vi "lock-in input sweep - T dependent.vi"() -> ()   [LabVIEW 2022 SP3]
uses:
  <vilib>/Utility/file.llb/Write To Spreadsheet File (DBL).vi
panel:
  out "phase":dbl=-1.07289e-06
  in  "Parameter (1: X) 2":u16(ring)=2 items=["X"=1, "Y"=2, "R"=3, "Theta"=4, "Channel 1"=5, "Channel 2"=6, "Aux In 1"=7, "Aux In 2"=8, "Aux In 3"=9, "Aux In 4"=10]
  in  "auto phase":bool
  in  "manual phase":dbl
  in  "harm#2":dbl=1.0
  out "loop run":i32=1
  in  "loop #":i32=1
  in  "Save data or not":bool=TRUE
  in  "path (folder + filename)":string="D:\\test"
  in  "Clear Plot":bool
  out "XY Graph":cluster{dbl[], dbl[]}(graph)={[0.0, 0.020000000000000018, 0.040000000000000036, 0.05999999999999994, 0.07999999999999996, 0.09999999999999998, 0.12, 0.14, 0.16000000000000003, 0.17999999999999994, 0.19999999999999996, 0.21999999999999997, 0.24, 0.26, 0.28, 0.29999999999999993, 0.31999999999999995, 0.33999999999999997, 0.36, 0.38, 0.4, 0.42000000000000004, 0.43999999999999995, 0.45999999999999996, 0.48, 0.5, 0.52, 0.54, 0.56, 0.5800000000000001, 0.6, 0.62, 0.64, 0.6599999999999999, 0.6799999999999999, 0.7, 0.72, 0.74, 0.76, 0.78, 0.8, 0.8200000000000001, 0.84, 0.86, 0.88, 0.9, 0.92, 0.94, 0.96, 0.98, 1.0, 0.98, 0.96, 0.94, 0.9199999999999999, 0.9000000000000001, 0.8800000000000001, 0.8600000000000001, 0.8400000000000001, 0.8200000000000001, 0.8, 0.78, 0.76, 0.74, 0.72, 0.7, 0.6799999999999999, 0.6600000000000001, 0.6400000000000001, 0.6200000000000001, 0.6000000000000001, 0.5800000000000001, 0.56, 0.54, 0.52, 0.5, 0.48, 0.45999999999999996, 0.43999999999999995, 0.41999999999999993, 0.40000000000000013, 0.3800000000000001, 0.3600000000000001, 0.3400000000000001, 0.32000000000000006, 0.30000000000000004, 0.28, 0.26, 0.24, 0.21999999999999997, 0.19999999999999996, 0.17999999999999994, 0.15999999999999992, 0.14000000000000012, 0.1200000000000001, 0.10000000000000009, 0.08000000000000007, 0.06000000000000005, 0.040000000000000036, 0.020000000000000018, 0.0, 0.020000000000000018, 0.040000000000000036, 0.05999999999999994, 0.07999999999999996, 0.09999999999999998, 0.12, 0.14, 0.16000000000000003, 0.17999999999999994, 0.19999999999999996, 0.21999999999999997, 0.24, 0.26, 0.28, 0.29999999999999993, 0.31999999999999995, 0.33999999999999997, 0.36, 0.38, 0.4, 0.42000000000000004, 0.43999999999999995, 0.45999999999999996, 0.48, 0.5, 0.52, 0.54, 0.56, 0.5800000000000001, 0.6, 0.62, 0.64, 0.6599999999999999, 0.6799999999999999, 0.7, 0.72, 0.74, 0.76, 0.78, 0.8, 0.8200000000000001, 0.84, 0.86, 0.88, 0.9, 0.92, 0.94, 0.96, 0.98, 1.0, 0.98, 0.96, 0.9400000000000001, 0.92, 0.9, 0.88, 0.86, 0.84, 0.8200000000000001, 0.8, 0.78, 0.76, 0.74, 0.72, 0.7000000000000001, 0.68, 0.66, 0.64, 0.62, 0.6, 0.58, 0.56, 0.54, 0.52, 0.5, 0.48, 0.46, 0.44, 0.42, 0.4, 0.38, 0.36, 0.34, 0.32, 0.3, 0.28, 0.26, 0.24, 0.22, 0.2, 0.18, 0.16, 0.14, 0.12, 0.1, 0.08, 0.06, 0.04, 0.02, 0.0, 0.0, 0.19999999999999996, 0.3999999999999999, 0.6, 0.8, 1.0, 0.8, 0.6000000000000001, 0.40000000000000013, 0.20000000000000018, 0.0, 0.19999999999999996, 0.3999999999999999, 0.6, 0.8, 1.0, 0.8, 0.6000000000000001, 0.4, 0.2, 0.0, 0.0, 0.19999999999999996, 0.3999999999999999, 0.6, 0.8, 1.0, 0.8, 0.6000000000000001, 0.40000000000000013, 0.20000000000000018, 0.0, 0.19999999999999996, 0.3999999999999999, 0.6, 0.8, 1.0, 0.8, 0.6000000000000001, 0.4, 0.2, 0.0, 0.0], [-2.3842e-07, -3.5763e-07, -2.3842e-07, -1.1921e-07, 0.0, 0.0, 0.0, 1.1921e-07, 1.1921e-07, 3.5763e-07, 5.9605e-07, 5.9605e-07, 5.9605e-07, 4.76841e-07, 3.5763e-07, 1.1921e-07, 1.1921e-07, 1.1921e-07, 3.5763e-07, 3.5763e-07, 2.3842e-07, 1.1921e-07, -1.1921e-07, -3.5763e-07, -5.9605e-07, -4.76841e-07, -3.5763e-07, -2.3842e-07, 0.0, 0.0, 0.0, -2.3842e-07, -2.3842e-07, -1.1921e-07, -2.3842e-07, -2.3842e-07, -2.3842e-07, -2.3842e-07, -3.5763e-07, -2.3842e-07, -2.3842e-07, -2.3842e-07, -3.5763e-07, -2.3842e-07, -1.1921e-07, 0.0, 1.1921e-07, 0.0, 0.0, -1.1921e-07, -1.1921e-07, 0.0, 0.0, 0.0, 0.0, 0.0, 0.0, 0.0, -1.1921e-07, -2.3842e-07, -3.5763e-07, -3.5763e-07, -3.5763e-07, -2.3842e-07, -2.3842e-07, 0.0, 2.3842e-07, 3.5763e-07, 3.5763e-07, 2.3842e-07, 2.3842e-07, 2.3842e-07, 3.5763e-07, 5.9605e-07, 5.9605e-07, 7.15259e-07, 8.34469e-07, 8.34469e-07, 5.9605e-07, 1.1921e-07, -1.1921e-07, -2.3842e-07, -2.3842e-07, -1.1921e-07, 0.0, 1.1921e-07, 1.1921e-07, 0.0, 0.0, 1.1921e-07, 2.3842e-07, 3.5763e-07, 3.5763e-07, 2.3842e-07, 2.3842e-07, 1.1921e-07, -1.1921e-07, -2.3842e-07, -3.5763e-07, -4.76841e-07, -4.76841e-07, -4.76841e-07, -3.5763e-07, -3.5763e-07, -2.3842e-07, -2.3842e-07, -1.1921e-07, 0.0, 1.1921e-07, 2.3842e-07, 3.5763e-07, 2.3842e-07, 0.0, -2.3842e-07, -3.5763e-07, -3.5763e-07, -3.5763e-07, -2.3842e-07, -1.1921e-07, -1.1921e-07, 0.0, 1.1921e-07, 1.1921e-07, 1.1921e-07, 0.0, 0.0, -1.1921e-07, 0.0, -1.1921e-07, -1.1921e-07, -1.1921e-07, -1.1921e-07, -2.3842e-07, -1.1921e-07, 1.1921e-07, 2.3842e-07, 1.1921e-07, 0.0, -1.1921e-07, -3.5763e-07, -3.5763e-07, -3.5763e-07, -2.3842e-07, -2.3842e-07, 0.0, 1.1921e-07, 2.3842e-07, 2.3842e-07, 1.1921e-07, -1.1921e-07, -2.3842e-07, -3.5763e-07, -4.76841e-07, -7.15259e-07, -7.15259e-07, -7.15259e-07, -7.15259e-07, -4.76841e-07, -2.3842e-07, -2.3842e-07, -2.3842e-07, -3.5763e-07, -4.76841e-07, -4.76841e-07, -4.76841e-07, -3.5763e-07, -3.5763e-07, -2.3842e-07, -1.1921e-07, 1.1921e-07, 2.3842e-07, 3.5763e-07, 4.76841e-07, 5.9605e-07, 7.15259e-07, 7.15259e-07, 7.15259e-07, 5.9605e-07, 1.1921e-07, -1.1921e-07, -2.3842e-07, -2.3842e-07, -2.3842e-07, -2.3842e-07, -2.3842e-07, 0.0, 1.1921e-07, 2.3842e-07, 1.1921e-07, 0.0, -2.3842e-07, -2.3842e-07, -2.3842e-07, -2.3842e-07, -1.1921e-07, 0.0, -1.1921e-07, -1.1921e-07, -1.1921e-07, 0.0, 1.1921e-07, -2.3842e-07, -2.3842e-07, -2.3842e-07, -2.3842e-07, -2.3842e-07, -1.1921e-07, -1.1921e-07, 0.0, 0.0, 1.1921e-07, 1.1921e-07, 2.3842e-07, 2.3842e-07, 2.3842e-07, 2.3842e-07, 1.1921e-07, 0.0, -2.3842e-07, -2.3842e-07, -2.3842e-07, -2.3842e-07, -1.1921e-07, -1.1921e-07, -1.1921e-07, -2.3842e-07, -2.3842e-07, -3.5763e-07, -3.5763e-07, -4.76841e-07, -4.76841e-07, -4.76841e-07, -4.76841e-07, -4.76841e-07, -4.76841e-07, -4.76841e-07, -3.5763e-07, -3.5763e-07, -2.3842e-07, 0.0, 0.0, 1.1921e-07, 1.1921e-07, -4.76841e-07]}
  out "para1 Measurement":dbl=-2.3842e-07
  in  "Parameter (1: X)":u16(ring)=1 items=["X"=1, "Y"=2, "R"=3, "Theta"=4, "Channel 1"=5, "Channel 2"=6, "Aux In 1"=7, "Aux In 2"=8, "Aux In 3"=9, "Aux In 4"=10]
  out "gate voltage":dbl format="%#_13g"
  in  "GATE STEP(mv)":i32=20
  in  "GATE Low Value (default 0)":dbl
  in  "GATE High Value":dbl=1.0
  in  "lovkin waiting":dbl=0.2 format="%#_13g"
  in  "frequency":dbl=50.0 format="%#_13g"
  in  "Input Connection (0: Single-Ended Voltage)":u16(ring)=1 items=["Single-Ended Voltage", "Differential Voltage", "1 MOhm Current Gain", "100 MOhm Current Gain"]
  in  "LOCKIN address":refnum<visa-resource-name>="GPIB0::10::INSTR"
  # "Lock-in"
  # "top Gate Setting"
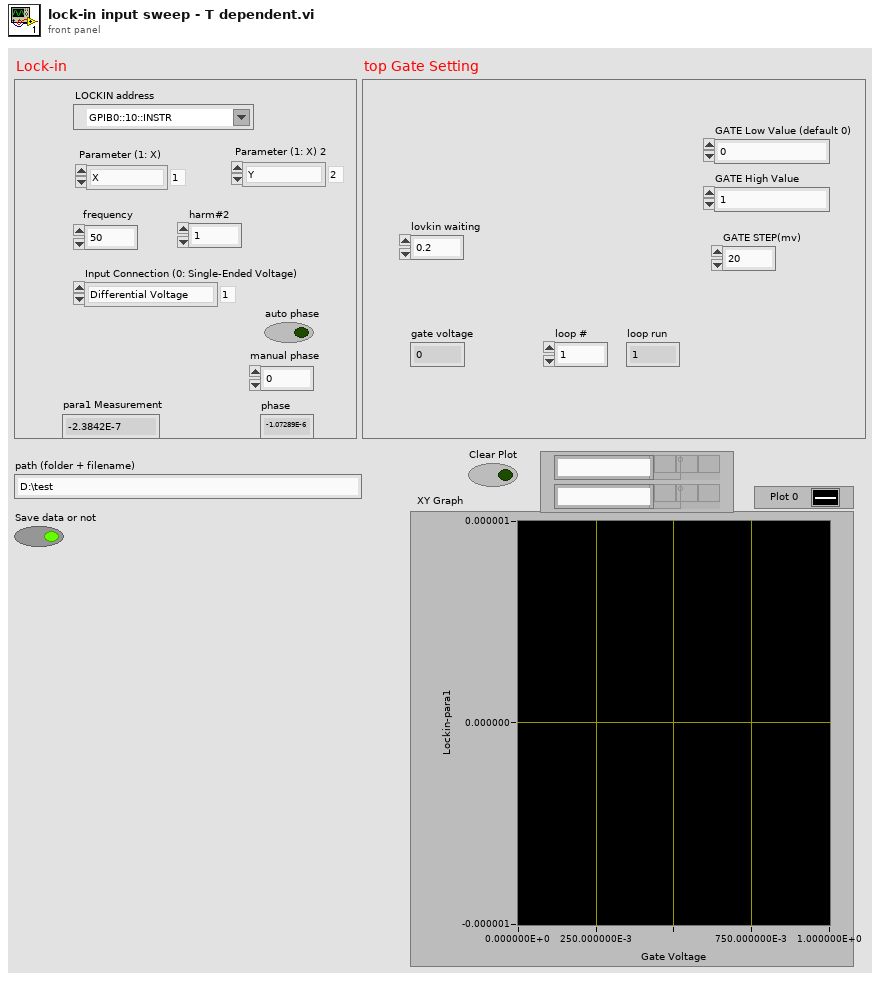
[diagram p1: front panel]
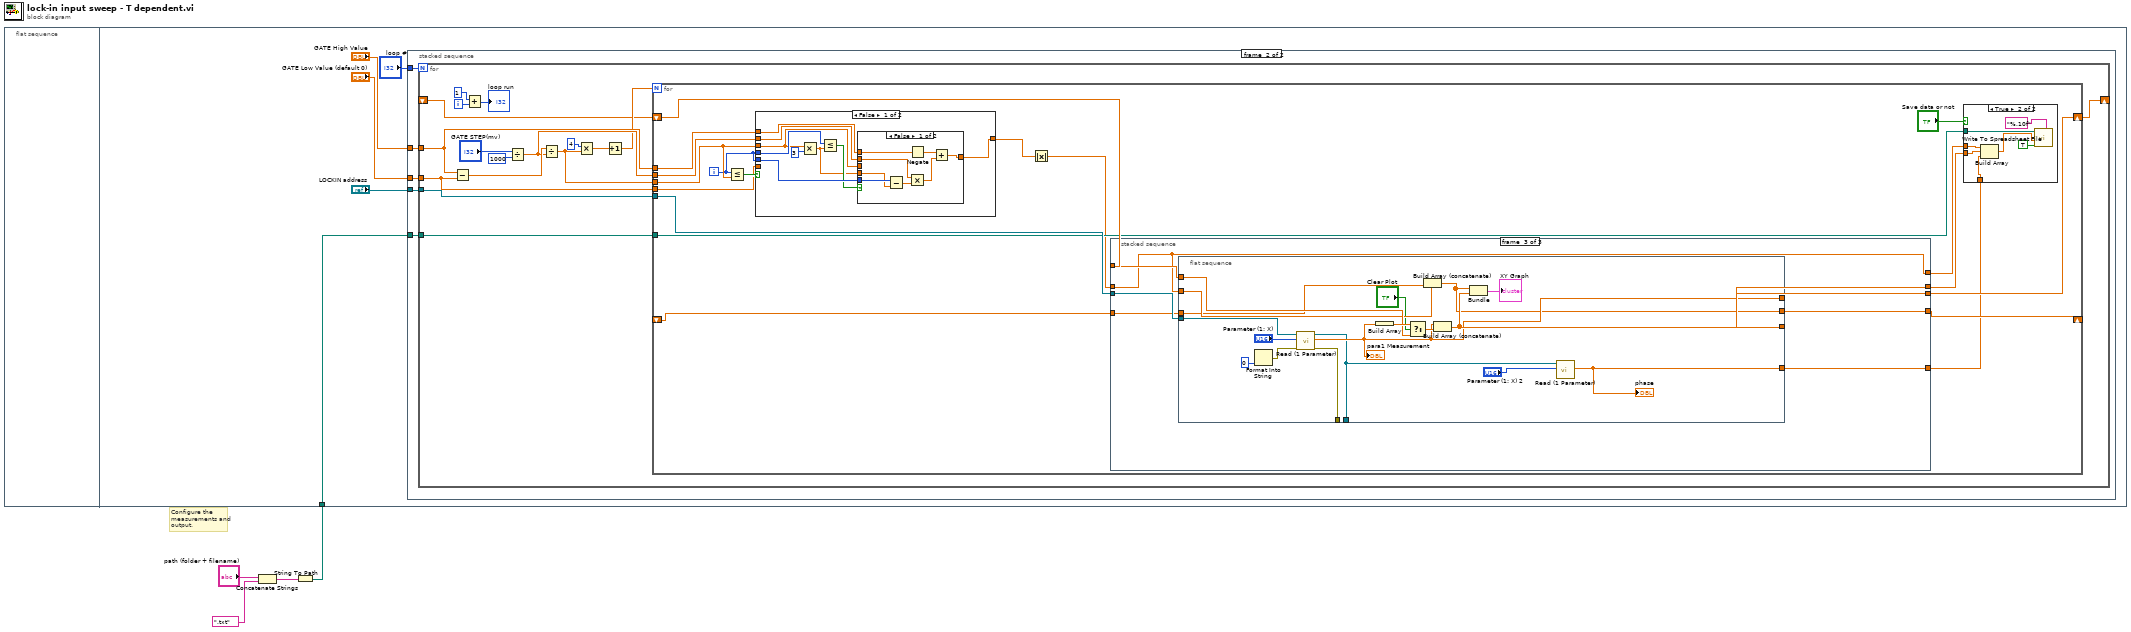
[diagram p0: block diagram]
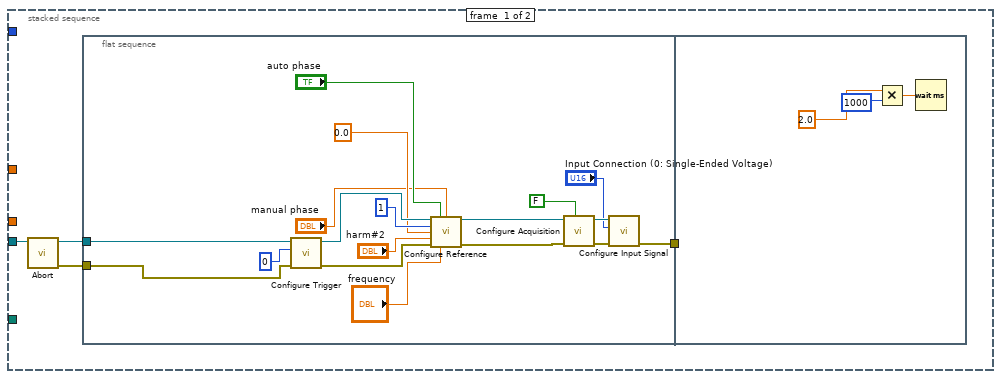
[diagram p2: hidden frame]
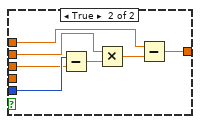
[diagram p4: hidden frame]
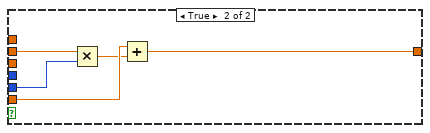
[diagram p5: hidden frame]
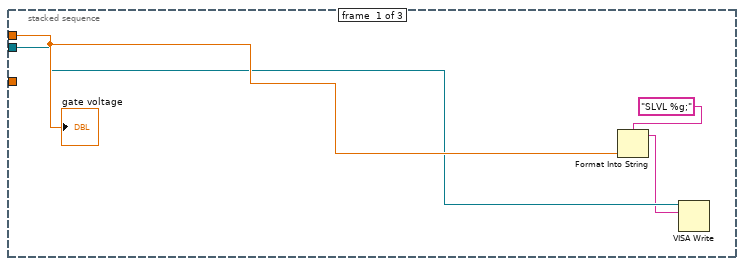
[diagram p6: hidden frame]
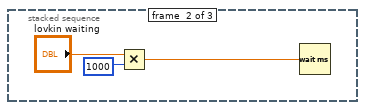
[diagram p7: hidden frame]
diagram:
  # "Configure the measurements and output."
  n1 = flat-sequence {
    tunnel: w1 -> [w6]
    frame #0 {
    }
    frame #1 {
      n2 = stacked-sequence {
        tunnel: "LOCKIN address" -> [w12 w39]
        tunnel: "GATE High Value" -> [_ w37]
        tunnel: "GATE Low Value (default 0)" -> [_ w38]
        tunnel: w6 -> [_ w36]
        tunnel: "loop #" -> [_ w35]
        frame #0 {
          n3 = call <instrlib>:"Abort.vi"("VISA resource name"=w12) -> ("error out"=w10:errorcluster, "VISA resource name out"=w11:refnum<visa-resource-name>)  [unwired: 9 in]
          n4 = flat-sequence {
            tunnel: w11 -> [w31]
            tunnel: [w16] -> w13
            tunnel: w10 -> [w15]
            tunnel: w13 -> [_]
            frame #0 {
              n5 = call <instrlib>:"Configure Trigger.vi"("error in (no error)"=w15, "Trigger Source (0: Internal)"=0, "VISA resource name"=w31) -> ("error out"=w25:errorcluster, "VISA resource name out"=w26:refnum<visa-resource-name>)  [unwired: 7 in]
              n6 = call <instrlib>:"Configure Reference.vi"("VISA resource name"=w26, "Auto Phase (T: Enabled)"="auto phase", "Manual Phase (0 Degree)"="manual phase", "Reference Source (1: Internal)"=1, "Sine Output Amplitude (1 V)"=0.0 ("Sine Output Amplitude (1 V) 2"), "Detection Harmonic Number (1)"="harm#2", "error in (no error)"=w25, "Internal Reference Frequency (1000 Hz)"="frequency") -> ("VISA resource name out"=w23:refnum<visa-resource-name>, "error out"=w18:errorcluster)  [unwired: 6 in]
              n7 = call <instrlib>:"Configure Acquisition.vi"("Continuous Storage (T: Enable)"=FALSE, "error in (no error)"=w18, "VISA resource name"=w23) -> ("error out"=w17:errorcluster, "VISA resource name out"=w21:refnum<visa-resource-name>)  [unwired: 7 in]
              n8 = call <instrlib>:"Configure Input Signal.vi"("error in (no error)"=w17, "Input Connection (0: Single-Ended Voltage)"="Input Connection (0: Single-Ended Voltage)", "VISA resource name"=w21) -> ("error out"=w16:errorcluster)  [unwired: 7 in, 1 out]
            }
            frame #1 {
              n9 = Multiply(x=2.0 ("SD stabilization(S) 2"), y=1000) -> (x*y=w34:dbl)
              n10 = Wait (ms)(milliseconds to wait=w34) -> ()  [unwired: 1 out]
            }
          }
        }
        frame #1 {
          n11 = for {
            N: w35 -> [_]
            tunnel: w39 -> [w56]
            tunnel: w38 -> [w50]
            tunnel: w37 -> [w49]
            tunnel: w36 -> [w48]
            shift-right: [w44] -> _
            shift-left: _ -> [w43]
            i -> [w41]
            n12 = Subtract(x=w49, y=w50) -> (x-y=w52:dbl)
            n13 = Add(x=1, y=w41) -> (x+y=→"loop run":i32)
            n14 = Divide(x="GATE STEP(mv)", y=1000) -> (x/y=w51:dbl)
            n15 = Divide(x=w52, y=w51) -> (x/y=w47:dbl)
            n16 = Multiply(x=4, y=w47) -> (x*y=w46:dbl)
            n17 = Increment(x=w46) -> (x+1=w45:dbl)
            n18 = for {
              N: w45 -> [_]
              tunnel: w56 -> [w74]
              tunnel: w51 -> [w69]
              shift-right: [w72] -> w44
              shift-left: w43 -> [w73]
              tunnel: w47 -> [w67]
              tunnel: w50 -> [w70]
              tunnel: w49 -> [w68]
              tunnel: w48 -> [w63]
              shift-right: [w61] -> _
              shift-left: _ -> [w60]
              i -> [w66]
              n19 = Less Or Equal?(x=w66, y=w67) -> (x <= y?=w71:bool)
              n20 = case shown="False" w71 {
                tunnel: w70 -> [_ w110]
                tunnel: w66 -> [w90 w109]
                tunnel: w69 -> [w89 w108]
                tunnel: [w87 w106] -> w59
                tunnel: w68 -> [w88 _]
                tunnel: w67 -> [w83 _]
                tunnel: w66 -> [w86 _]
                frame False {
                  n21 = Multiply(x=w83, y=3) -> (x*y=w82:dbl)
                  n22 = Less Or Equal?(x=w86, y=w82) -> (x <= y?=w84:bool)
                  n23 = case shown="False" w84 {
                    tunnel: w90 -> [w98 w105]
                    tunnel: w89 -> [w96 w103]
                    tunnel: w88 -> [w92 w101]
                    tunnel: [w94 w100] -> w87
                    tunnel: w83 -> [_ w99]
                    tunnel: w82 -> [w91 _]
                    frame False {
                      n24 = Subtract(x=w98, y=w91) -> (x-y=w97:dbl)
                      n25 = Multiply(x=w96, y=w97) -> (x*y=w95:dbl)
                      n26 = Negate(x=w92) -> (-x=w93:dbl)
                      n27 = Add(x=w93, y=w95) -> (x+y=w94:dbl)
                    }
                    frame True {
                      n28 = Subtract(x=w105, y=w99) -> (x-y=w104:dbl)
                      n29 = Multiply(x=w103, y=w104) -> (x*y=w102:dbl)
                      n30 = Subtract(x=w101, y=w102) -> (x-y=w100:dbl)
                    }
                  }
                }
                frame True {
                  n31 = Multiply(x=w108, y=w109) -> (x*y=w107:dbl)
                  n32 = Add(x=w110, y=w107) -> (x+y=w106:dbl)
                }
              }
              n33 = Absolute Value(x=w59) -> (abs(x)=w58:dbl)
              n34 = stacked-sequence {
                tunnel: w74 -> [w112 _ w123]
                tunnel: w58 -> [w113 _ w121]
                tunnel: w73 -> [_ _ w125]
                tunnel: [_ _ w124] -> w72
                tunnel: [_ _ w122] -> w65
                tunnel: [_ _ w121] -> w64
                tunnel: [_ _ w120] -> w61
                tunnel: w60 -> [_ _ w119]
                tunnel: [_ _ w118] -> w57
                frame #0 {
                  n35 = Format Into String(format string="SLVL %g;", w113) -> (resulting string=w111:string)  [unwired: 2 in, 1 out]
                  n36 = VISA Write(VISA resource name=w112, write buffer=w111) -> ()  [unwired: 1 in, 3 out]
                  "gate voltage" <- w113
                }
                frame #1 {
                  n37 = Multiply(x="lovkin waiting", y=1000) -> (x*y=w117:dbl)
                  n38 = Wait (ms)(milliseconds to wait=w117) -> ()  [unwired: 1 out]
                }
                frame #2 {
                  n39 = flat-sequence {
                    tunnel: w125 -> [w137]
                    tunnel: w123 -> [w135]
                    tunnel: w121 -> [w133]
                    tunnel: [w127] -> _
                    tunnel: [w132] -> _
                    tunnel: [w136] -> w124
                    tunnel: [w134] -> w122
                    tunnel: [w130] -> w120
                    tunnel: w119 -> [w129]
                    tunnel: [w126] -> w118
                    frame #0 {
                      n40 = Format Into String(0) -> (error out=w143:errorcluster)  [unwired: 3 in, 1 out]
                      n41 = call <instrlib>:"Read (1 Parameter).vi"("error in (no error)"=w143, "Parameter (1: X)"="Parameter (1: X)", "VISA resource name"=w135) -> ("error out"=w132:errorcluster, "Measurement"=w134:dbl, "VISA resource name out"=w127:refnum<visa-resource-name>)  [unwired: 6 in]
                      "para1 Measurement" <- w134
                      n42 = Build Array(w134) -> (w140:dbl[])
                      n43 = Select(t=w140, s="Clear Plot", f=w137) -> (s? t:f=w141:dbl[])
                      n44 = Build Array (concatenate)(w133, w129) -> (w130:dbl[])
                      n45 = Build Array (concatenate)(w134, w141) -> (w136:dbl[])
                      n46 = Bundle(w130, w136) -> (→"XY Graph":cluster{dbl[], dbl[]})  [unwired: 1 in]
                      n47 = call <instrlib>:"Read (1 Parameter).vi"("Parameter (1: X)"="Parameter (1: X) 2", "VISA resource name"=w127) -> ("Measurement"=w126:dbl)  [unwired: 7 in, 2 out]
                      "phase" <- w126
                    }
                  }
                }
              }
              n48 = case shown="True" "Save data or not" {
                tunnel: w65 -> [_ w81]
                tunnel: w64 -> [_ w80]
                tunnel: w63 -> [_ w78]
                tunnel: w57 -> [_ w75]
                frame False {
                }
                frame True {
                  n49 = Build Array(w80, w81, w75) -> (w79:dbl[])
                  n50 = call-poly <vilib>:"Write To Spreadsheet File.vi"("format (%.3f)"="%.10f", "append to file? (new file:F)"=TRUE, "1D data"=w79, "file path (dialog if empty)"=w78) -> ()  [unwired: 4 in, 1 out]
                }
              }
            }
          }
        }
      }
    }
  }
  n51 = Concatenate Strings("path (folder + filename)", ".txt") -> (w2:string)
  n52 = String To Path(string=w2) -> (path=w1:path)
